vi "Set DataCell.vi"   [LabVIEW 2016, in "DataGrid.lvlib" / "DataTable.lvclass"]
uses:
  <userlib>/LabVIEWdotNetDataGrid/source/DataTable/DataTable.lvclass
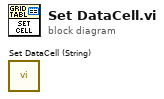
[diagram p0: block diagram]
diagram:
  n1 = call <userlib>:"Set DataCell (String).vi"() -> ()  [unwired: 14 in, 2 out]
